vi "testBenchmarkSystemDefinitionFails.vi"(8 "error in (no error)":errorcluster, 11 "TestCase in":refnum<class "VeriStandTestCaseTests.lvclass">) -> (0 "error out":errorcluster, 3 "TestCase out":refnum<class "VeriStandTestCaseTests.lvclass">)   [LabVIEW 2015, in "VeriStandTestCaseTests.lvclass"]
uses:
  VeriStandTestCaseTests.lvclass
  VeriStandTestCase.lvclass
  <vilib>/addons/_JKI Toolkits/VI Tester/TestCase.llb/TestCase.lvclass
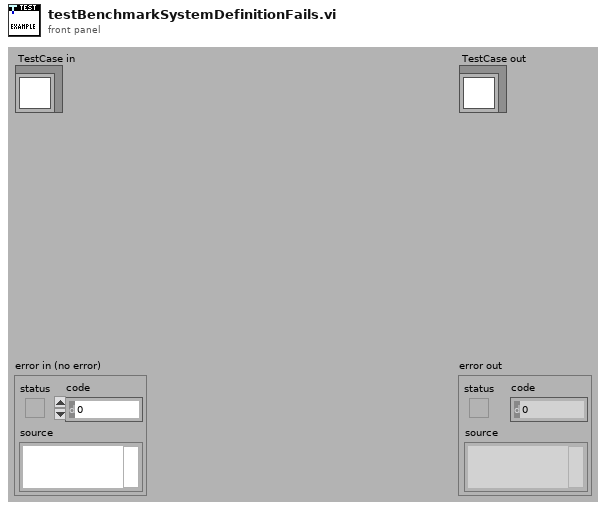
[diagram p1: front panel]
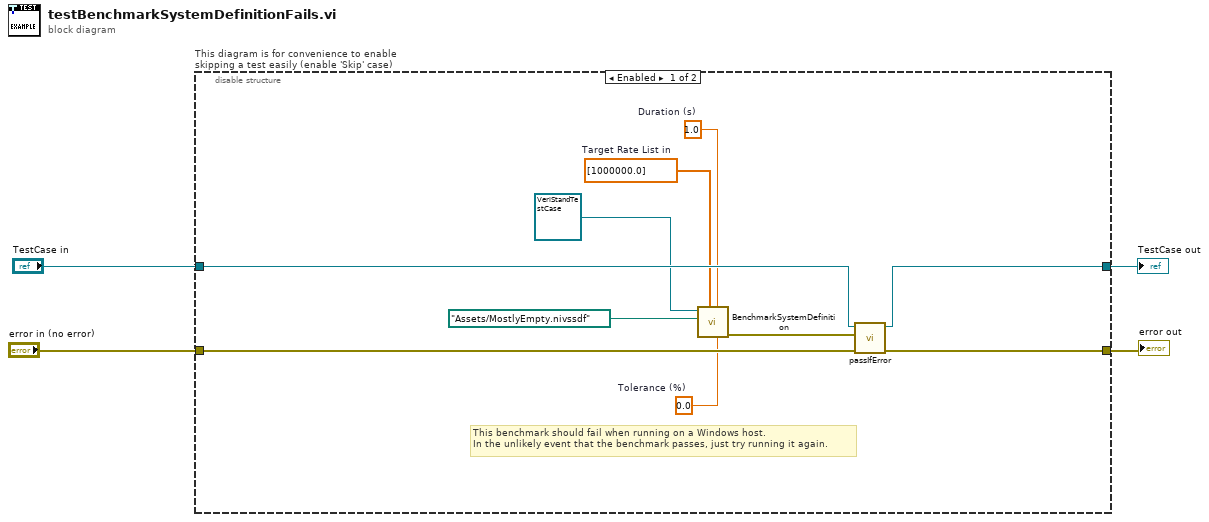
[diagram p0: block diagram]
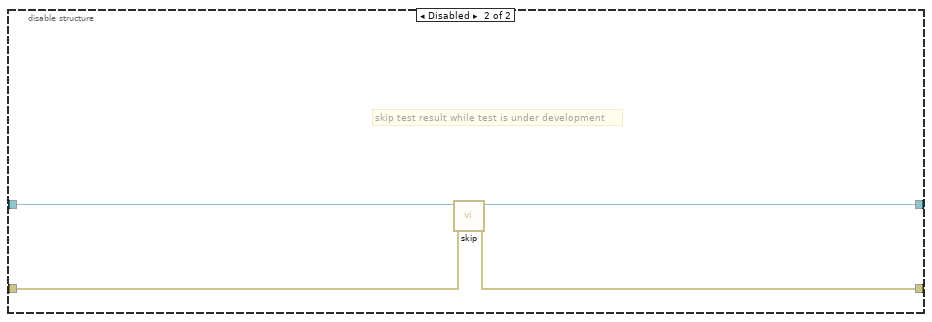
[diagram p2: hidden frame]
diagram:
  n1 = disable-structure "This diagram is for convenience to enable skipping a test easily (enable 'Skip' case)" shown="Enabled" {
    disable-tunnel: "TestCase in" -> [w12 w18]
    disable-tunnel: [w11 w16] -> w1
    disable-tunnel: [w13 w17] -> w3
    disable-tunnel: "error in (no error)" -> [w14 w15]
    frame Enabled {
      w5 = 0.0  # Tolerance (%)
      w6 = 1.0  # Duration (s)
      w7 = dbl[] [1000000.0]  # Target Rate List in
      # "This benchmark should fail when running on a Windows host.\nIn the unlikely event that the benchmark passes, just try running it again."
      n2 = call-dynamic "BenchmarkSystemDefinition.vi"("Tolerance (%)"=w5, "Duration (s)"=w6, "Target Rate List in"=w7, "System Definition File"=path "Assets/MostlyEmpty.nivssdf", "VeriStandTestCase in"=refnum<class "VeriStandTestCase.lvclass"> refnum ("VeriStand Test Case in")) -> ("error out"=w10:errorcluster)  [unwired: 5 in, 1 out]
      n3 = call-dynamic "passIfError.vi"("error in (no error)"=w14, "error"=w10, "TestCase in"=w12) -> ("error out"=w13:errorcluster, "TestCase out"=w11:refnum<class "VeriStandTestCaseTests.lvclass">)  [unwired: 7 in]
    }
    frame Disabled {
      # "skip test result while test is under development"
      n4 = call <vilib>:"skip.vi"("error in (no error)"=w15, "TestCase in"=w18) -> ("error out"=w17:errorcluster, "TestCase out"=w16:refnum<class "VeriStandTestCaseTests.lvclass">)  [unwired: 8 in]
    }
  }
  "error out" <- w3
  "TestCase out" <- w1
